vi "plusminuspoly.vi"   [LabVIEW 2017]
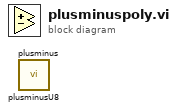
[diagram p0: block diagram]
diagram:
  n1 = call "plusminusU8.vi"() -> ()  [unwired: 6 in, 2 out]
  n2 = call "plusminus.vi"() -> ()  [unwired: 6 in, 2 out]
